vi "2_Waveform_Signal_Regression(Inference).vi"() -> ()   [LabVIEW 2020]
uses:
  <vilib>/Ngene/Deep Learning Toolkit/Toolkit/NN_Network/Controls/NN_Save_Before_Destroy_Options.ctl
  <vilib>/Ngene/Deep Learning Toolkit/Toolkit/NN_Network/API/NN_Set_Input/1D/NN_Set_Input(1D_SGL_idx).vi
  <vilib>/Ngene/Deep Learning Toolkit/Toolkit/Deep_Learning_Toolkit_by_Ngene.lvlib
  <vilib>/measure/NI_MABase.lvlib
panel:
  out "Frequency Chart":cluster{"Numeric Control":sgl, "Frequency":dbl}(graph)={"Numeric Control"=56.031754, "Frequency"=55.34351145038168}
  out "Predicted Frequency":sgl=56.031754 format="%#_3g"
  in  "Noise":dbl(slide)=1.6412213740458015 scale=0.0..5.0
  in  "Offset":dbl(slide) scale=-10.0..10.0
  out "Generated WaveForm":waveform(dbl)(graph)={"t0"=timestamp(0 s since 1904-01-01), "dt"=0.001, "Y"=[3.7335949831664412, -1.0099743489502353, -1.9601771660048801, -4.382936408985187, -4.816097724870346, -6.583531995677057, -8.054271525171744, -5.085783236554927, -5.537147311507594, -0.8453518413399739, 0.715670510634112, 3.048327868712305, 5.217820741905053, 5.723994129212894, 4.775150971924527, 7.648389392264417, 6.014393424084391, 4.821132599029929, 0.8200975613694901, 0.06425091357028431, -0.5456811974124045, -3.204587519648251, -5.52550808944998, -7.030077599482109, -7.382393857851424, -7.114872051215278, -5.638892707029925, -1.9977039901337714, -0.8903039981956059, 0.40142415695212175, 5.4046580783344496, 3.924860917429527, 7.437694272609867, 6.143915307071466, 4.729026777179259, 3.5616197282452227, 3.6481852372520995, 0.18543932800016516, -2.0959160042338443, -3.1406370124170033, -4.588788744340724, -5.494554060301203, -7.35574001894291, -5.412127823549914, -3.3991105867342957, -4.109746278334667, 1.0762185257166192, 2.107732141465938, 4.495502410220782, 5.367566211603192, 7.8777722702525015, 5.817264384911035, 5.0011218320392645, 3.6748160249604434, 3.275963328788425, 0.4582725201541183, -0.28807830553216096, -4.117816204399569, -6.015076744152964, -7.6059370845907495, -5.565384317687261, -4.815653595733104, -5.5712574431143915, -3.762788222123458, 0.6860717460049546, 3.069347222532093, 3.5063414022712545, 4.928445342108747, 5.900673043562946, 6.804915440654601, 7.157394950045802, 3.4351202900623274, 1.2463986783252894, 1.9667958453809593, -2.997567266277758, -5.208373987403888, -6.679735732236605, -6.993399576836023, -7.044695670672874, -6.001539322984119, -3.7101195958421456, -3.576656922097999, -1.4120168519678624, 2.2301785740913624, 2.691053631081544, 5.416834973871209, 6.586119103226053, 4.979718930392515, 4.545819443887861, 5.004809224878579, 2.1880802570067597, 0.30516492951160257, -2.7748202189591895, -4.451936293423629, -6.319981146614995, -6.896722445827438, -6.264433543069051, -6.663525858548047, -5.878036308437827, -2.2914812294675357]}
  in  "Phase":dbl(slide)=159.38931297709925 scale=0.0..360.0
  in  "Signal Type":T1(ring)
  in  "Amplitude":dbl(slide)=6.523664122137405 scale=0.1..10.0
  in  "Frequency":dbl(slide)=55.34351145038168 scale=10.0..100.0
  in  "Weight File Path":path=path "D:/Ngene/GitHub/deepltk_examples/2_Waveform_Processing/22_Waveform_Signal_Regression/working/WF_Regression/WF_Regression_weights_23_10_05__17_35_42.bin"
  in  "Network Configuration File Path":path=path "D:/Ngene/GitHub/deepltk_examples/2_Waveform_Processing/22_Waveform_Signal_Regression/working/WF_Regression/WF_Regression_net_cfg_23_10_05__17_35_42.cfg"
  in  "Stop":bool
  # "Overview: Demonstrates the usage of DeepLTK for loading the model pretrained for waveform signal regression (signal frequency prediction) and running for inference.\nRequirements: DeepLTK - Deep Learning Toolkit for LabVIEW (https://www.ngene.co/deep-learning-toolkit-for-labview)\nInstructions:\n1. Provide Network Configuration File Path and Weight File Path generated from training example.\n2. Run the VI\n3. Input Waveform parameters and observe the predicted frequency against reference value.\n4. Press the Stop button to stop the VI.\n\nMore Examples:  https://github.com/ngenehub/deepltk_examples"
  # "Waveform Signal Regression (Frequency Predictions) Inference"
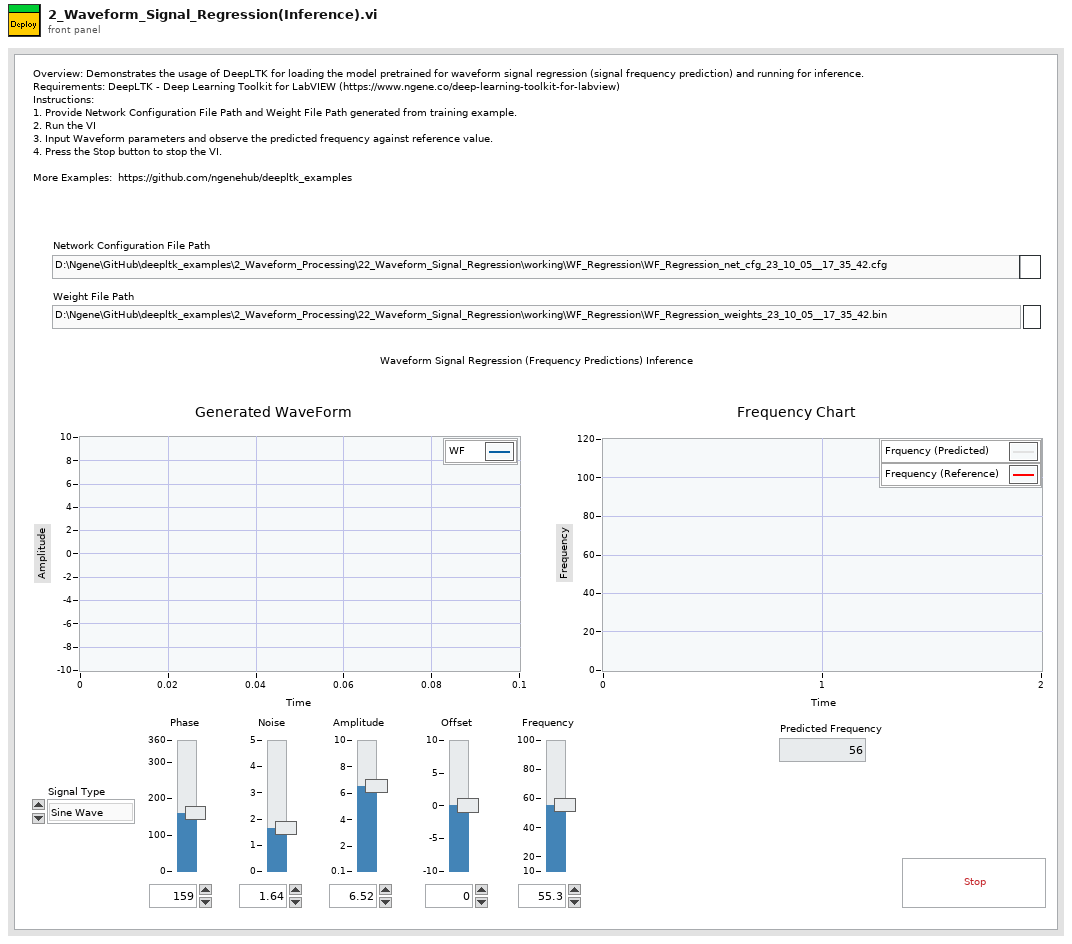
[diagram p1: front panel]
types:
  T1 = enum16{"Sine Wave", "Triangle Wave", "Square Wave", "Sawtooth Wave"}
  T2 = typedef "Deep_Learning_Toolkit_by_Ngene.lvlib/NN_Save_Before_Destroy_Options.ctl" = cluster{"CFG?":bool, "Weights?":bool, "Render?":bool}
  T3 = typedef "Deep_Learning_Toolkit_by_Ngene.lvlib/NN_Config_Params.ctl" = cluster{"Name":string, "mBatch":i32, "NN_Train_Params":T4, "LR_Decay_Policy":T7, "Labels":string[], "Loss":T9, "Max_WS_Size(B)":i64, "DryRun?":bool}
  T4 = typedef "Deep_Learning_Toolkit_by_Ngene.lvlib/NN_Train_Params.ctl" = cluster{"Optimizer":T5, "Beta_1":sgl, "Beta_2":sgl, "Weight Decay(L1)":sgl, "Weight Decay(L2)":sgl, "Data_Sampling":T6}
  T5 = typedef "Deep_Learning_Toolkit_by_Ngene.lvlib/NN_Train_Optimizer.ctl" = enum16{"SGD", "Adam", "Adagrad", "Adadelta", "RMSProp", "Nesterov"}
  T6 = typedef "Deep_Learning_Toolkit_by_Ngene.lvlib/NN_Train_Data_Sampling.ctl" = enum16{"Random", "Sequential"}
  T7 = typedef "Deep_Learning_Toolkit_by_Ngene.lvlib/NN_LR_Policy_Cfg.ctl" = cluster{"Policy_Type":T8, "LR0":dbl, "k":sgl, "WarmUp_Policy":enum16{"Step", "Ramp"}, "WarmUp_Iter":i32, "WarmUp_Ratio":sgl}
  T8 = typedef "Deep_Learning_Toolkit_by_Ngene.lvlib/NN_LR_Policy_Type.ctl" = enum16{"Manual", "Step", "Exp", "1/t"}
  T9 = typedef "Deep_Learning_Toolkit_by_Ngene.lvlib/NN_Loss_Config_Params.ctl" = cluster{"Loss_Type":T10, "Loss_Conf_Params":variant}
  T10 = typedef "Deep_Learning_Toolkit_by_Ngene.lvlib/NN_Loss_Type.ctl" = enum16{"None", "MSE", "CrossEntropy", "YOLO_v2", "YOLO_v4"}
  T11 = typedef "Deep_Learning_Toolkit_by_Ngene.lvlib/NN_Layer_Config_Params.ctl" = cluster{"Layer_Type":T12, "Layer_Conf_Params":variant, "Input Layers":string[]}
  T12 = typedef "Deep_Learning_Toolkit_by_Ngene.lvlib/NN_Layer_Type.ctl" = enum16{"Input1D", "Input3D", "Conv1D", "Conv2D", "Conv2D_Adv", "MaxPool", "AvgPool", "UpSample", "DropOut3D", "ShortCut", "Concat", "SoftMax3D", "FC", "DropOut", "Softmax", "Flatten", "YOLO_v2", "YOLO_v4", "Activation", "BatchNormalization", "LayerNormalization", "Scale", "Unsupported"}
  T13 = typedef "Deep_Learning_Toolkit_by_Ngene.lvlib/NN.ctl" = cluster{"Name":string, "No of Layers":i32, "mBatch":i32, "Layers":T14[], "Dimty":T15, "Dims_In":T16, "Dims_Out":T16, "Working_Dir":path, "Train?":bool, "Train_Params":T4, "LR_Update_Policy":T7, "Session Data":T17, "Ground_truth":T18, "NNg_hdls":T19, "NN_Device":T20, "GPU Id":i32, "Labels":string[], "Loss_Type":T10, "Loss_Cfg_Prms":variant, "NNG_WS":T21, "DryRun?":bool}
  T14 = typedef "Deep_Learning_Toolkit_by_Ngene.lvlib/NN_Layer_ref.ctl" = refnum<file>
  T15 = typedef "Deep_Learning_Toolkit_by_Ngene.lvlib/NN_In_Out_Dim-ty.ctl" = enum8{"In1D_Out1D", "In3D_Out1D", "In3D_Out3D", "In3D_OutBBox"}
  T16 = typedef "Deep_Learning_Toolkit_by_Ngene.lvlib/NN_Dims(C,H,W).ctl" = cluster{"C":i32, "H":i32, "W":i32}
  T17 = typedef "Deep_Learning_Toolkit_by_Ngene.lvlib/NN_Train_Session_Data.ctl" = cluster{"Epochs":sgl, "Tot_Iter":i32, "LR":sgl, "LR_iter":i32}
  T18 = typedef "Deep_Learning_Toolkit_by_Ngene.lvlib/NN_Ground_truth.ctl" = cluster{"Y":variant}
  T19 = typedef "Deep_Learning_Toolkit_by_Ngene.lvlib/nng_cuda_handles.ctl" = cluster{"cudnn":u64, "cublas":u64, "stream":u64, "curand":u64}
  T20 = typedef "Deep_Learning_Toolkit_by_Ngene.lvlib/NN_Device.ctl" = enum16{"CPU", "GPU"}
  T21 = typedef "Deep_Learning_Toolkit_by_Ngene.lvlib/NNG_WS.ctl" = cluster{"NNG_WS_Mem":T22, "Max_WS_Size":i64}
  T22 = typedef "Deep_Learning_Toolkit_by_Ngene.lvlib/NNg_WS_Mem_DVR.ctl" = refnum<data-value>
  T23 = typedef "Deep_Learning_Toolkit_by_Ngene.lvlib/NN_Layer.ctl" = cluster{"Name":string, "Layer_Data":T24, "Layer_Type":T12, "Dims_In":T16, "Layers_In":T14[], "Dims_Out":T16, "Layers_Out":T14[], "Metrics":T25, "GPU_Data":T26, "mBatch":i32, "NN_Device":T20, "NNg_hdls":T19, "Train?":bool, "Dimty":T27, "RecptField":T28, "Idx":i32}
  T24 = typedef "Deep_Learning_Toolkit_by_Ngene.lvlib/NN_Layer_Data_Refnum.ctl" = refnum<file>
  T25 = typedef "Deep_Learning_Toolkit_by_Ngene.lvlib/NN_Layer_Metrics.ctl" = cluster{"Data":dbl, "Params":dbl, "Ops":dbl}
  T26 = typedef "Deep_Learning_Toolkit_by_Ngene.lvlib/NNg_Layer_Data_Refnum.ctl" = refnum<file>
  T27 = typedef "Deep_Learning_Toolkit_by_Ngene.lvlib/NN_Layer_Dimty.ctl" = enum16{"1D", "3D"}
  T28 = typedef "Deep_Learning_Toolkit_by_Ngene.lvlib/NN_Layer_RF_State.ctl" = cluster{"Dims":T29, "J":T29}
  T29 = typedef "Deep_Learning_Toolkit_by_Ngene.lvlib/NN_Dims(V,H).ctl" = cluster{"V":i32, "H":i32}
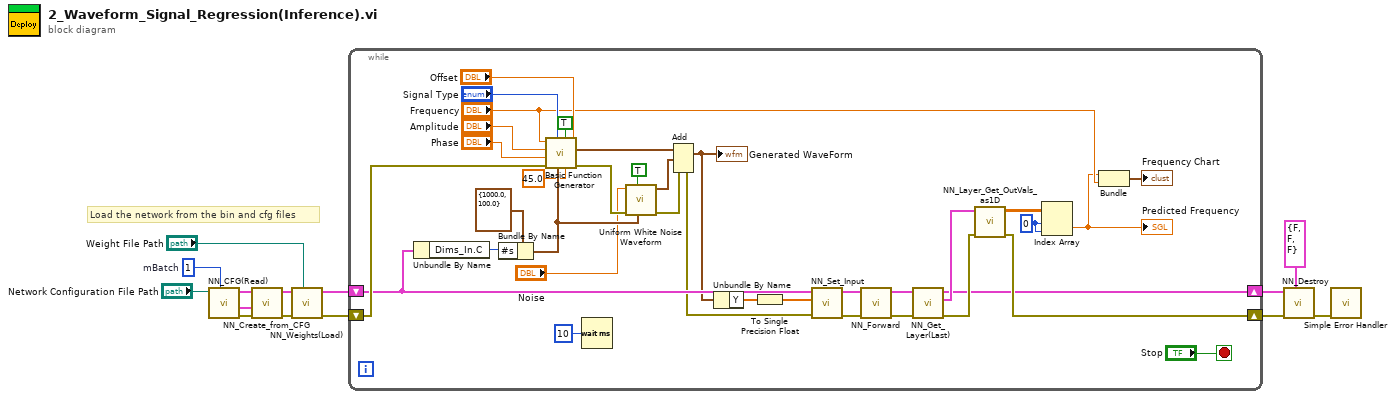
[diagram p0: block diagram]
diagram:
  w1 = 1  # mBatch
  # "Load the network from the bin and cfg files"
  n1 = call <vilib>:"NN_CFG(Read).vi"("mBatch"=w1, "CFG file path"="Network Configuration File Path") -> ("error out"=w8:errorcluster, "Net_Cfg"=w9:T3, "Layer_Cfg"=w7:T11[])  [unwired: 7 in]
  n2 = call <vilib>:"NN_Create_from_CFG.vi"("error in (no error)"=w8, "Net_Cfg"=w9, "Layer_Cfg"=w7) -> ("error out"=w11:errorcluster, "NN out"=w6:T13)  [unwired: 7 in]
  n3 = call <vilib>:"NN_Weights(Load).vi"("Weight File Path"="Weight File Path", "error in (no error)"=w11, "NN in"=w6) -> ("error out"=w5:errorcluster, "NN out"=w4:T13)  [unwired: 7 in]
  n4 = while {
    shift-right: [w49] -> w14
    shift-left: w5 -> [w50]
    shift-right: [w32] -> w13
    shift-left: w4 -> [w34]
    stop <- "Stop" stop-if-true
    w29 = 0 ("index (row)")
    n5 = Unbundle By Name(w34) -> ("Dims_In.C"=w33:i32)
    n6 = Bundle By Name(cluster=cluster{"Fs":dbl, "#s":dbl} {"Fs"=1000.0, "#s"=100.0} ("sampling info"), "#s"=w33) -> (w26:cluster{"Fs":dbl, "#s":dbl})
    n7 = call <vilib>:"Basic Function Generator.vi"("offset"="Offset", "square wave duty cycle (%)"=45.0, "reset signal"=TRUE, "sampling info"=w26, "signal type"="Signal Type", "error in (no error)"=w50, "phase"="Phase", "amplitude"="Amplitude", "frequency"="Frequency") -> ("error out"=w27:errorcluster, "signal out"=w30:waveform(dbl))  [unwired: 1 out]
    n8 = Wait (ms)(milliseconds to wait=u32 10) -> ()  [unwired: 1 out]
    n9 = call <vilib>:"Uniform White Noise Waveform.vi"("sampling info"=w26, "reset signal"=TRUE, "error in (no error)"=w27, "amplitude"="Noise") -> ("error out"=w23:errorcluster, "signal out"=w24:waveform(dbl))  [unwired: 6 in]
    n10 = Add(1:w24, 2:w30, 4:w23) -> (0:w25:waveform(dbl), 3:w22:errorcluster)
    "Generated WaveForm" <- w25
    n11 = Unbundle By Name(w25) -> ("Y"=w40:dbl[])
    n12 = To Single Precision Float(number=w40) -> (single precision float=w15:sgl[])
    n13 = call-poly <vilib>:"NN_Set_Input.vi"("error in (no error)"=w22, "Data_In(1D_SGL)"=w15, "NN In"=w34) -> ("error out"=w48:errorcluster, "NN Out"=w45:T13)  [unwired: 7 in]
    n14 = call <vilib>:"NN_Forward.vi"("error in (no error)"=w48, "NN in"=w45) -> ("error out"=w47:errorcluster, "NN out"=w46:T13)  [unwired: 6 in, 2 out]
    n15 = call <vilib>:"NN_Get_Layer(Last).vi"("error in (no error)"=w47, "NN in"=w46) -> ("error out"=w44:errorcluster, "Last_Layer"=w43:T23, "NN out"=w32:T13)  [unwired: 6 in, 1 out]
    n16 = call <vilib>:"NN_Layer_Get_OutVals_as1D.vi"("error in (no error)"=w44, "Layer"=w43) -> ("error out"=w49:errorcluster, "Out(as1D)"=w42:sgl[][])  [unwired: 8 in]
    n17 = Index Array(array=w42, index (row)=w29, index (col)=w29) -> (element=w16:sgl)
    "Predicted Frequency" <- w16
    n18 = Bundle("Numeric Control"=w16, "Frequency"="Frequency") -> (→"Frequency Chart":cluster{"Numeric Control":sgl, "Frequency":dbl})  [unwired: 1 in]
  }
  n19 = call <vilib>:"NN_Destroy.vi"("Save (T, T, T)"=T2 {"CFG?"=FALSE, "Weights?"=FALSE, "Render?"=FALSE}, "error in (no error)"=w14, "NN in"=w13) -> ("error out"=w2:errorcluster)  [unwired: 7 in, 1 out]
  n20 = call <vilib>:"Simple Error Handler.vi"("error in (no error)"=w2) -> ()  [unwired: 4 in, 5 out]
